vi "LV SCISDK Read Custom Packet Data.vi"(0 "Path":string, 2 "handle":u64, 3 "error in (no error)":errorcluster) -> (7 "function return":i32, 8 "buffer out":T1, 9 "handle out":u64, 10 "error out":errorcluster)   [LabVIEW 2021, in "SciSDK_Labview.lvlib"]
doc: "SCISDKLABVIEW_DLL_API int LV_SCISDK_ReadData(char* Path, LV_OSCILLOSCOPE_DECODED_BUFFER* buffer, void* handle);"
uses:
  SciSDK_Labview.lvlib
  SciSDK_VC++/x64/Debug/SciSDK_Labview.dll
panel:
  out "data 2":cluster{"n":dbl, "data":dbl[]}[](array[cluster])
  in  "data":cluster{"n":u32, "data":u32[]}[](array[cluster])=[{"n"=0, "data"=[]}, {"n"=0, "data"=[]}, {"n"=0, "data"=[0, 0, 1]}]
  in  "buffer":T2
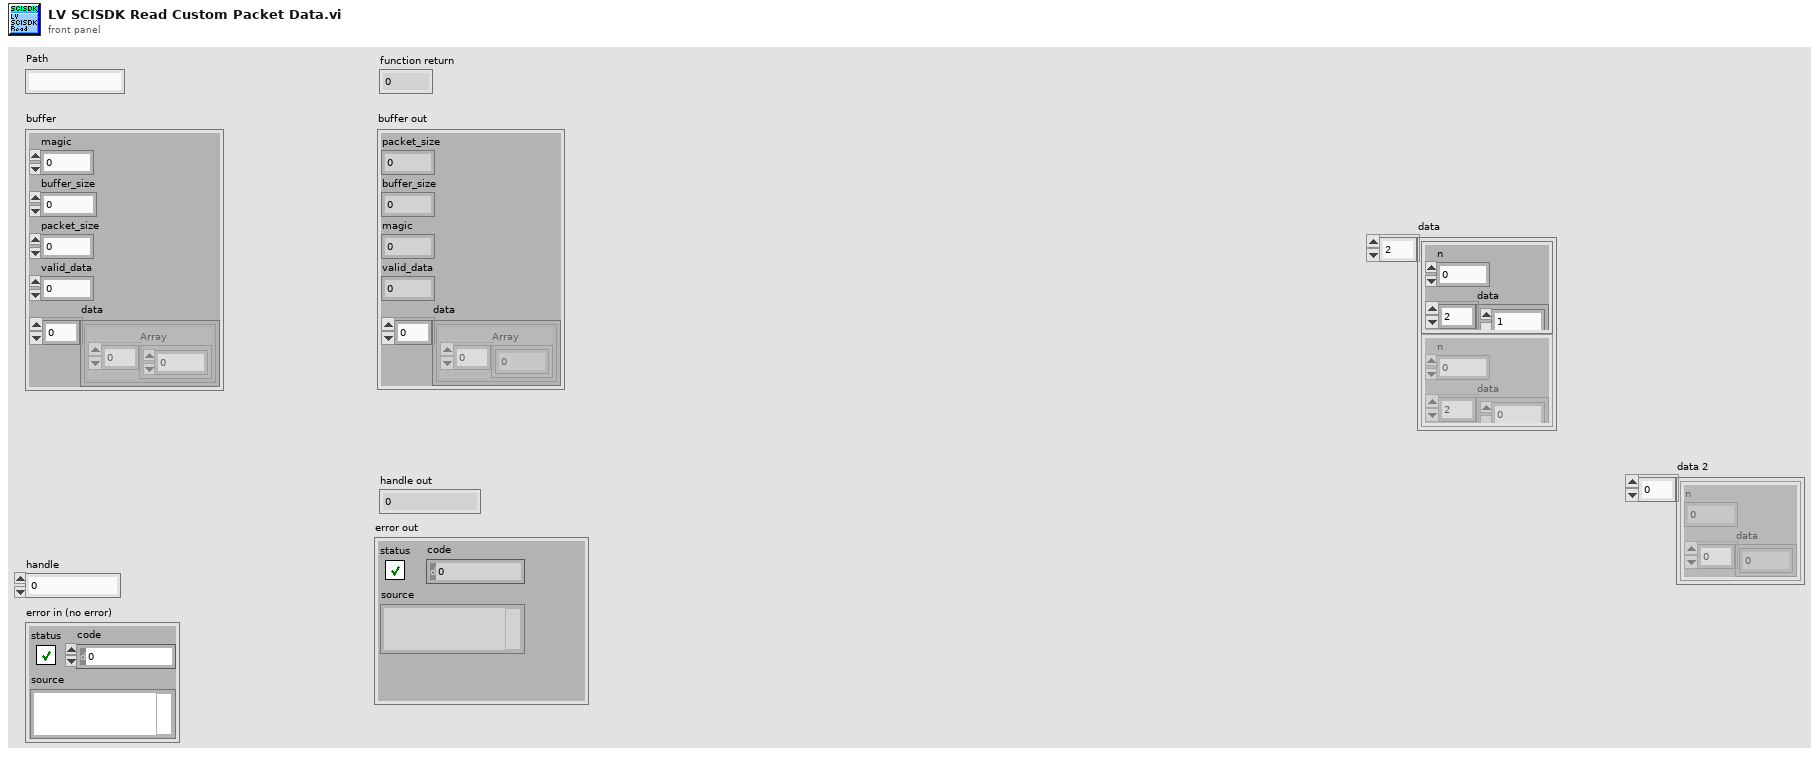
[diagram p1: front panel]
types:
  T1 = cluster{"packet_size":u32, "buffer_size":u32, "magic":u32, "valid_data":dbl, "data":cluster{"Array":dbl[]}[]}
  T2 = cluster{"magic":u32, "buffer_size":u32, "packet_size":u32, "valid_data":u32, "data":cluster{"Array":i32[]}[]}
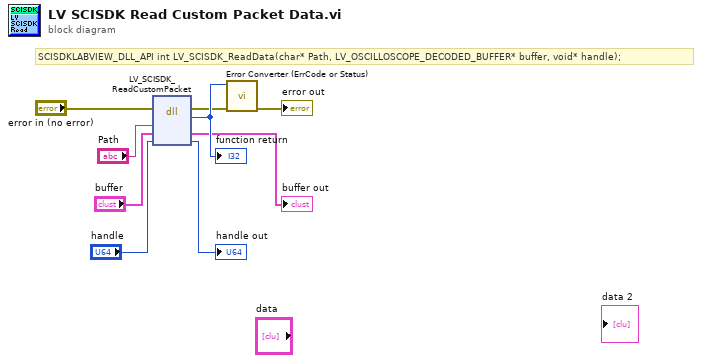
[diagram p0: block diagram]
diagram:
  # "SCISDKLABVIEW_DLL_API int LV_SCISDK_ReadData(char* Path, LV_OSCILLOSCOPE_DECODED_BUFFER* buffer, void* handle);"
  n1 = dll-call lib="C:/git/scisdk/SciSDK_VC++/x64/Debug/SciSDK_Labview.dll" fn="LV_SCISDK_ReadCustomPacket"(error in="error in (no error)", "Path"="Path", "buffer"="buffer", "handle"="handle") -> (error out=w4:errorcluster, "return type"=w9:i32, "buffer"=→"buffer out":T2, "handle"=→"handle out":u64)  [unwired: 3 in, 1 out]
  "function return" <- w9
  n2 = call <userlib>:"Error Converter (ErrCode or Status).vi"("error in (no error)"=w4, "error code"=w9) -> ("error out"=→"error out":errorcluster)  [unwired: 9 in]
